vi "Update Fluidic Para.vi"(8 "Error In":errorcluster, 11 "Fluidic Para":T1) -> (0 "Error Out":errorcluster)   [LabVIEW 2019, in "Fluidic Process.lvlib"]
uses:
  Fluidic Process.lvlib
  SubVI/Fluidic Para.ctl
  Queues/Queues.lvlib
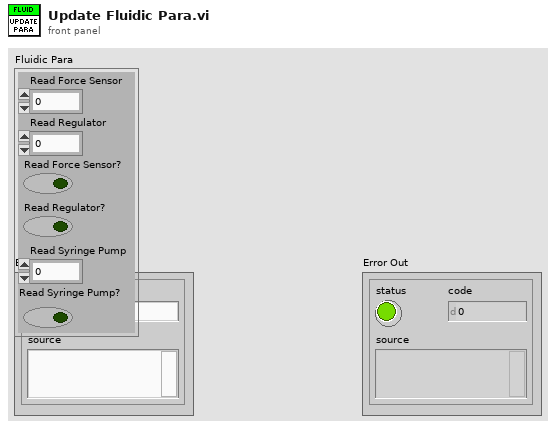
[diagram p1: front panel]
types:
  T1 = typedef "Fluidic Process.lvlib/Fluidic Para.ctl" = cluster{"Read Force Sensor":i32, "Read Regulator":i32, "Read Force Sensor?":bool, "Read Regulator?":bool, "Read Syringe Pump":i32, "Read Syringe Pump?":bool}
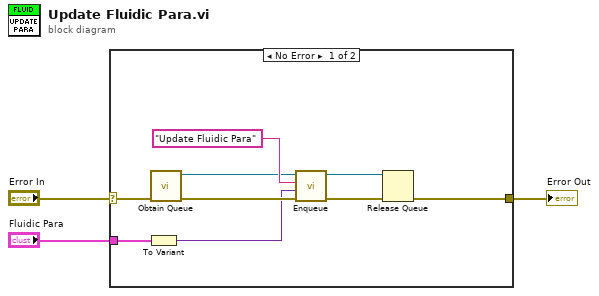
[diagram p0: block diagram]
diagram:
  n1 = case shown="No Error" "Error In" {
    selector: "Error In" -> [w8 w13]
    tunnel: [w9 w13] -> w3
    tunnel: "Fluidic Para" -> [w5 _]
    frame No Error {
      n2 = To Variant(anything=w5) -> (Variant=w4:variant)
      n3 = call "Obtain Queue.vi"("Error In"=w8) -> ("Error Out"=w7:errorcluster, "Queue out"=w6:refnum<queue>)  [unwired: 9 in]
      n4 = call "Enqueue.vi"("Error In"=w7, "Data"=w4, "State"="Update Fluidic Para", "Queue in"=w6) -> ("Error Out"=w11:errorcluster, "Queue out"=w10:refnum<queue>)  [unwired: 6 in]
      n5 = Release Queue(queue=w10, error in (no error)=w11) -> (error out=w9:errorcluster)  [unwired: 1 in, 2 out]
    }
    frame Error {
    }
  }
  "Error Out" <- w3
